vi "Do.vi"(8 "error in (no error)":errorcluster, 10 "Actor in":refnum<class "Actor.lvclass">, 11 "Notify Subscribers Msg":refnum<class "Notify Subscribers Msg.lvclass">) -> (0 "error out":errorcluster, 2 "Actor out":refnum<class "Actor.lvclass">)   [LabVIEW 2017, in "Mediator.lvlib" / "Notify Subscribers Msg.lvclass"]
doc: "This VI delivers the message to the actor by calling the appropriate method(s) on the actor.\n\n<License>\nCopyright © 2017 Composed Systems, LLC | All rights reserved\nwww.composed.io\n\nAuthor: Ethan Stern <ethan.stern@composed.io>\n\nThis software is provided \"AS IS\" WITHOUT WARRANTIES, either express or implied, AND IS FOR EDUCATIONAL PURPOSES ONLY.\n</License>"
uses:
  Notify Subscribers Msg.lvclass
  <vilib>/ActorFramework/Actor/Actor.lvclass
  Topic/Topic.lvclass
  C:/Program Files (x86)/National Instruments/LabVIEW 2017/vi.lib/ActorFramework/Actor/Actor.lvclass
  Notify Subscribers Msg.lvclass/Notify Subscribers Msg.ctl
  Topic/Topic.lvclass/Topic.ctl
  IMediator/PublishRequest/PublishRequest.lvclass/PublishRequest.ctl
  IMediator/ISubscriptionPolicy/ISubscriptionPolicy.lvclass/ISubscriptionPolicy.ctl
  Topic/Publish to List.vi
  IMediator/PublishRequest/Read Publisher ID.vi
  IMediator/ISubscriptionPolicy/Execute Subscription Policy.vi
  IMediator/ISubscriptionPolicy/ISubscriptionPolicy.lvclass
  IMediator/PublishRequest/PublishRequest.lvclass
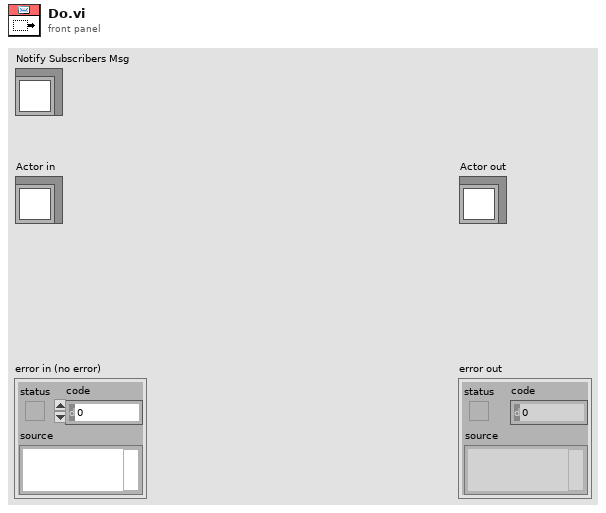
[diagram p1: front panel]
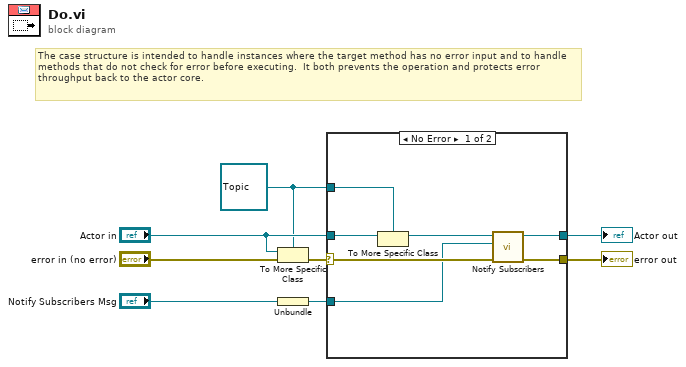
[diagram p0: block diagram]
diagram:
  w3 = refnum<class "Topic.lvclass"> refnum ("Actor in")
  # "The case structure is intended to handle instances where the target method has no error input and to handle methods that do not check for error before executing.  It both prevents the operation and protects error throughput back to the actor core."
  n1 = To More Specific Class(target class=w3, reference="Actor in", error in="error in (no error)") -> (error out=w2:errorcluster)  [unwired: 1 out]
  n2 = Unbundle("Notify Subscribers Msg") -> (w1:refnum<class "PublishRequest.lvclass">)
  n3 = case shown="No Error" w2 {
    selector: w2 -> [w13 w17]
    tunnel: [w15 w17] -> w8
    tunnel: [w14 w16] -> w7
    tunnel: "Actor in" -> [w12 w16]
    tunnel: w3 -> [w11 _]
    tunnel: w1 -> [w9 _]
    frame No Error {
      n4 = To More Specific Class(target class=w11, reference=w12) -> (specific class reference=w10:refnum<class "Topic.lvclass">)  [unwired: 1 in, 1 out]
      n5 = call "Notify Subscribers.vi"("error in (no error)"=w13, "PublishRequest"=w9, "Topic in"=w10) -> ("error out"=w15:errorcluster, "Topic out"=w14:refnum<class "Topic.lvclass">)  [unwired: 7 in]
    }
    frame Error {
      # "If type check fails, pass the\noriginal object out again."
    }
  }
  "error out" <- w8
  "Actor out" <- w7
